vi "PUMP RAMP 3 (SubVI).vi"(0 "Dynamic Data":dynamicdata(waveform), 5 "Numeric":i16, 7 "Seq in":dbl[][](array[numeric])=[[20.0, 60.0, 40.0], [60.0, 40.0, 20.0], [100.0, 100.0, 100.0]], 11 "Boolean":bool) -> (2 "Weight (S1)":dbl, 3 "target reached":i32, 4 "Time (s)":dbl, 6 "bal_previous":i32, 8 "Target (g)":dbl, 10 "Waveform Chart 2":dynamicdata(graph), 12 "Rate (g/s)":dbl, 13 "Step 2":i32, 14 "x/y":dbl)   [LabVIEW 2015]
uses:
  BERTTA.dll
panel:
  out "DAQ assistant (PAM i/o)":bool[](array[boolean])
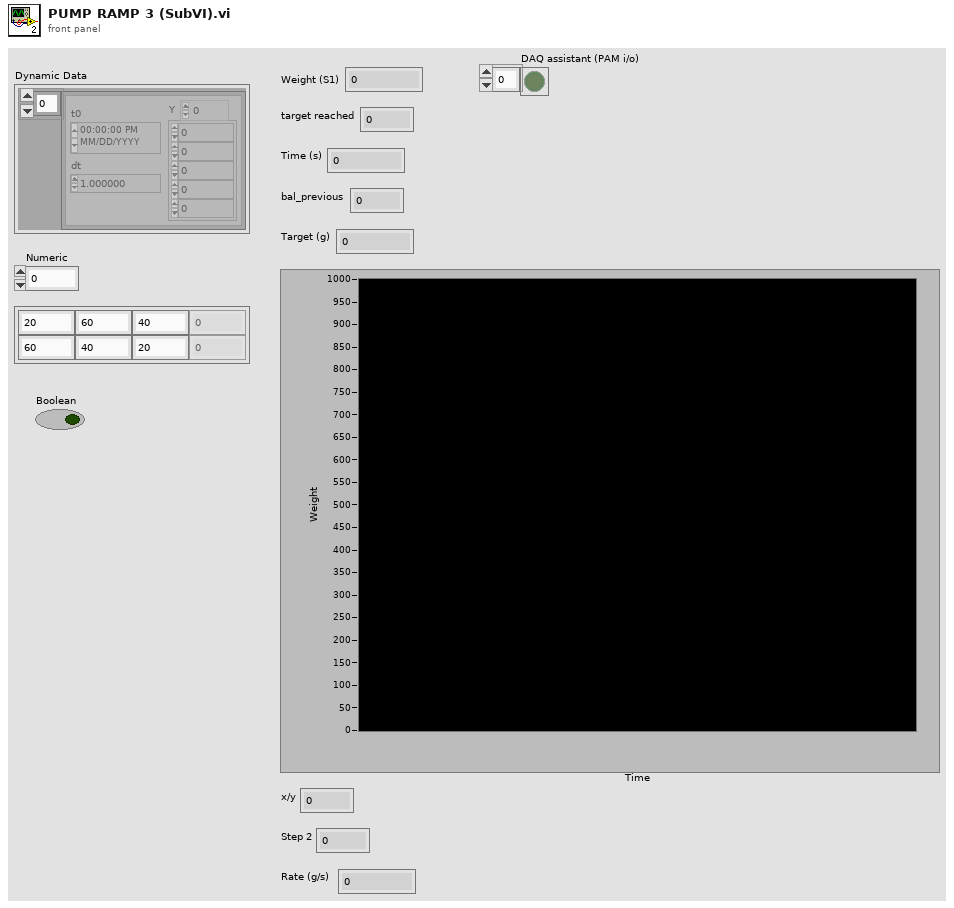
[diagram p1: front panel]
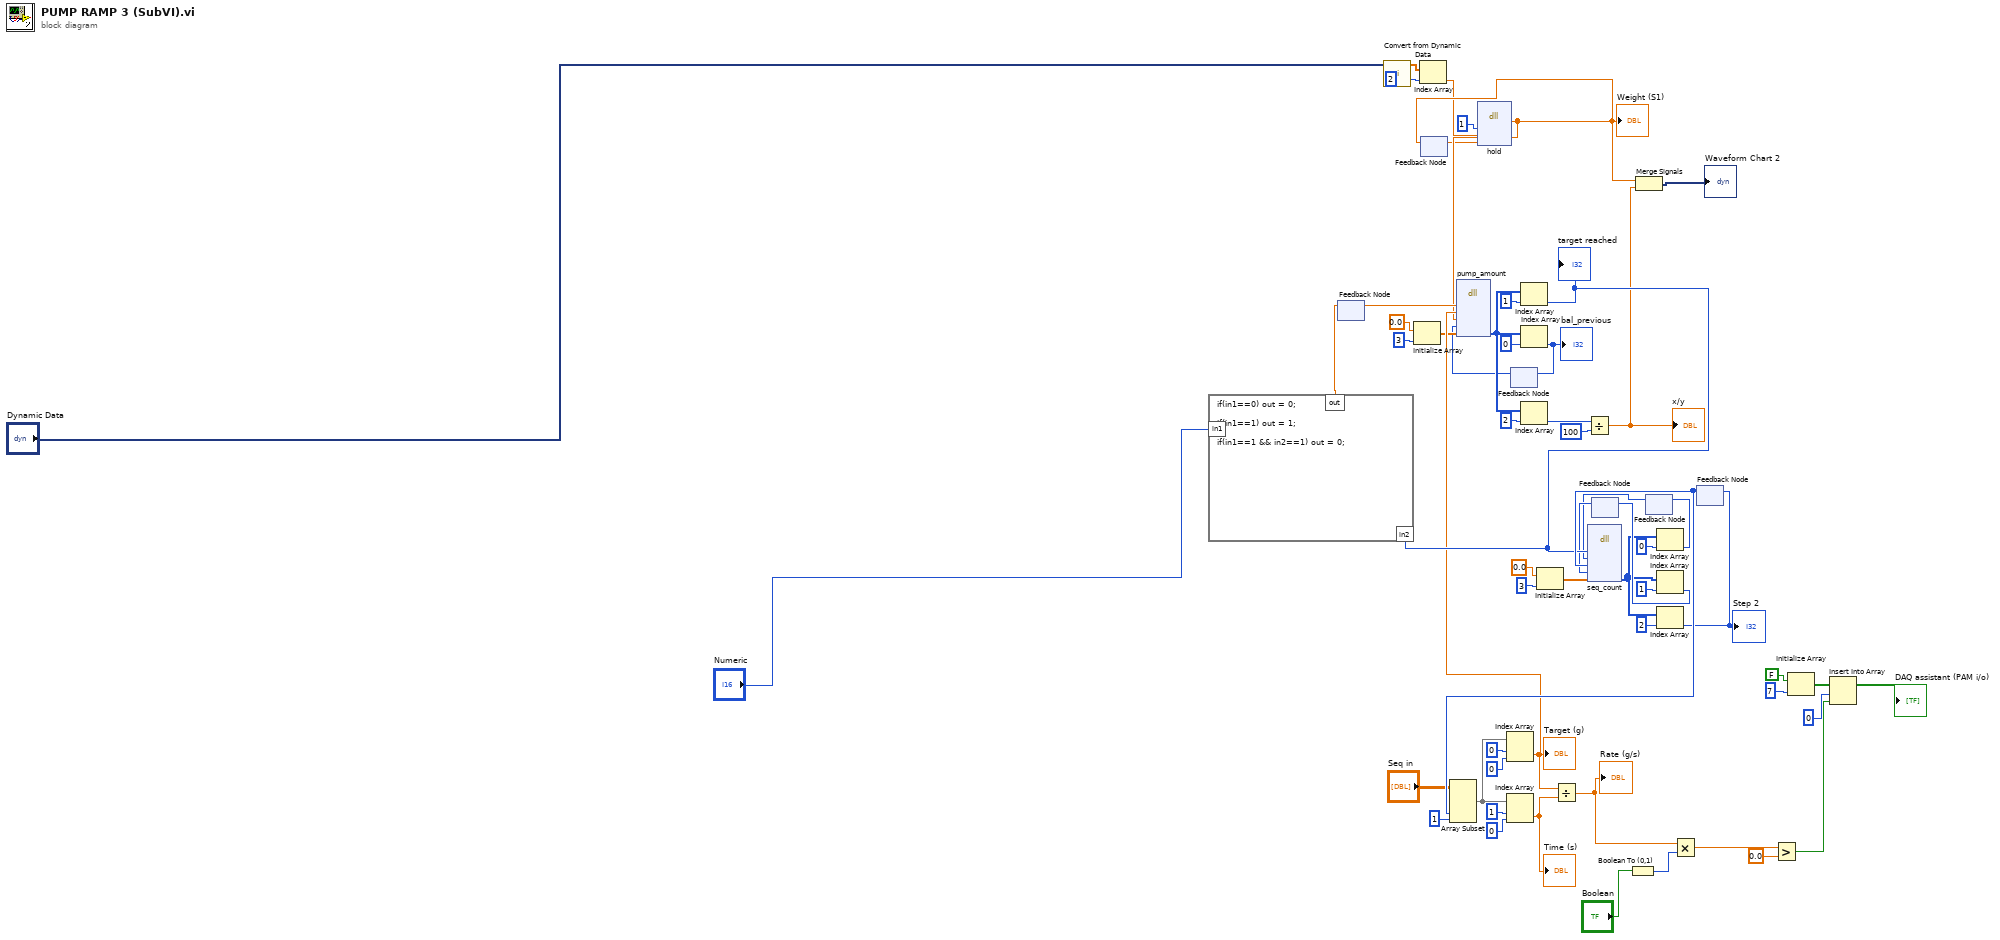
[diagram p0: block diagram]
diagram:
  n1 = feedback #1() -> (w54:dbl)  [unwired: 1 in]
  n2 = call "Convert from Dynamic Data"("Dynamic Data Type"="Dynamic Data") -> ("Array"=w21:dbl[])  [unwired: 3 in]
  n3 = Initialize Array(0.0 ("element"), 3 ("dimension size")) -> (w31:dbl[])
  n4 = Index Array(array=w21, index=2) -> (element=w22:dbl)
  n5 = feedback #2() -> (w23:dbl)  [unwired: 1 in]
  n6 = dll-call lib="C:/Users/xlaraser/Documents/Visual Studio 2017/Projects/Bertta/BERTTA/Debug/BERTTA.dll" fn="hold"("enable"=1, "in1"=w22, "in2"=w23) -> ("return type"=w34:dbl)  [unwired: 6 in, 2 out]
  "Weight (S1)" <- w34
  n7 = feedback-in #2(w34) -> ()
  n8 = feedback #3() -> (w28:i32)  [unwired: 1 in]
  n9 = Initialize Array(0.0 ("element"), 3 ("dimension size")) -> (w40:dbl[])
  n10 = feedback #4() -> (w48:i32)  [unwired: 1 in]
  n11 = Boolean To (0,1)(Boolean="Boolean") -> (0, 1=w3:i16)
  n12 = feedback #5() -> (w47:i32)  [unwired: 1 in]
  n13 = feedback #6() -> (w56:i32)  [unwired: 1 in]
  n14 = Array Subset(array="Seq in", index (col)=w56, length (col)=1 ("length")) -> (w15:dbl[][])  [unwired: 2 in]
  n15 = Index Array(array=w15, index (row)=0, index (col)=0 ("disabled index (col)")) -> (element=w36:dbl)
  "Target (g)" <- w36
  n16 = dll-call lib="C:/Users/xlaraser/Documents/Visual Studio 2017/Projects/Bertta/BERTTA/Debug/BERTTA.dll" fn="pump_amount"("enable"=w54, "target"=w36, "bal"=w34, "bal_previous"=w28, "params"=w31) -> ("params"=w33:i32[])  [unwired: 8 in, 2 out]
  n17 = Index Array(array=w15, index (row)=1, index (col)=0 ("disabled index (col)")) -> (element=w19:dbl)
  "Time (s)" <- w19
  n18 = Index Array(array=w33, index=1) -> (element=w52:i32)
  "target reached" <- w52
  n19 = formula code="if(in1==0) out = 0;\n\nif(in1==1) out = 1;\n\nif(in1==1 && in2==1) out = 0;"("in1"="Numeric", "in2"=w52) -> ("out"=w53:dbl)
  n20 = feedback-in #1(w53) -> ()
  n21 = Index Array(array=w33, index=0) -> (element=w27:i32)
  "bal_previous" <- w27
  n22 = feedback-in #3(w27) -> ()
  n23 = Index Array(array=w33, index=2) -> (element=w37:i32)
  n24 = Divide(x=w36, y=w19) -> (x/y=w2:dbl)
  "Rate (g/s)" <- w2
  n25 = Divide(x=w37, y=100) -> (x/y=w38:dbl)
  "x/y" <- w38
  n26 = dll-call lib="C:/Users/xlaraser/Documents/Visual Studio 2017/Projects/Bertta/BERTTA/Debug/BERTTA.dll" fn="seq_count"("in1"=w52, "in2"=w47, "in3"=w56, "in4"=w48, "params"=w40) -> ("params"=w46:i32[])  [unwired: 8 in, 2 out]
  n27 = Merge Signals(w34, w38) -> (→"Waveform Chart 2":dynamicdata)
  n28 = Index Array(array=w46, index=0) -> (element=w49:i32)
  n29 = feedback-in #5(w49) -> ()
  n30 = Index Array(array=w46, index=1) -> (element=w50:i32)
  n31 = feedback-in #4(w50) -> ()
  n32 = Index Array(array=w46, index=2) -> (element=w55:i32)
  "Step 2" <- w55
  n33 = Multiply(x=w2, y=w3) -> (x*y=w4:dbl)
  n34 = feedback-in #6(w55) -> ()
  n35 = Greater?(x=w4, y=0.0) -> (0:w5:bool)
  n36 = Initialize Array(FALSE ("element"), 7 ("dimension size")) -> (w9:bool[])
  n37 = Insert Into Array(array=w9, index=0, new element=w5) -> (→"DAQ assistant (PAM i/o)":bool[])
